vi "Monitoreo.vi"() -> ()   [LabVIEW 2020]
uses:
  <vilib>/Instr/_visa.llb/VISA Configure Serial Port (Instr).vi
panel:
  out "x+1":dbl
  out "concatenated string 2":string
  in  "string":string
  out "concatenated string":string
  in  "Boolean 2":bool
  in  "Boolean":bool
  in  "stop":bool
  in  "VISA resource name":refnum<visa-resource-name>
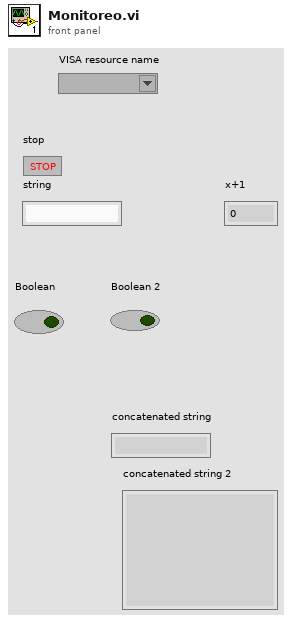
[diagram p1: front panel]
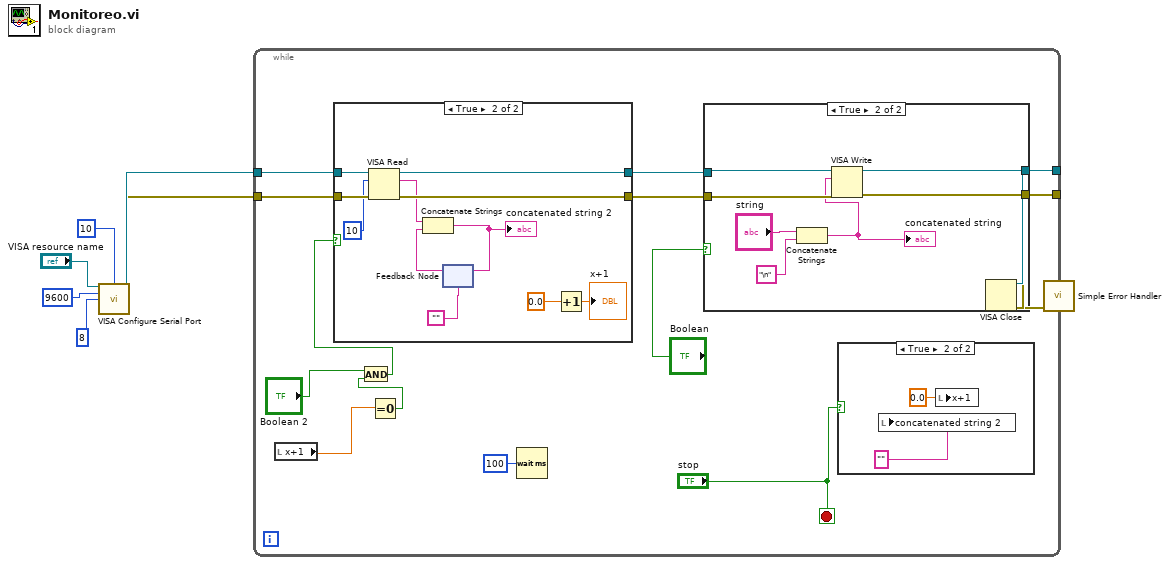
[diagram p0: block diagram]
diagram:
  n1 = call-poly "VISA Configure Serial Port"("VISA resource name"="VISA resource name", "termination char\n(0xA = '\\n' = LF)"=u8 10 ("termination char\n(0xA = '\\n' = LF)"), "baud rate (9600)"=u32 9600, "data bits (8)"=u16 8) -> ("VISA resource name out"=w7:refnum<visa-resource-name>, "error out"=w6:errorcluster)  [unwired: 10 in]
  n2 = while {
    tunnel: w7 -> [w22]
    tunnel: w6 -> [w17]
    tunnel: [w20] -> w5
    tunnel: [w18] -> w3
    stop <- "stop" stop-if-true
    n3 = local read "x+1"() -> (w13:dbl)
    n4 = Equal To 0?(x=w13) -> (x = 0?=w12:bool)
    n5 = And(x="Boolean 2", y=w12) -> (x .and. y?=w10:bool)
    n6 = case shown="True" w10 {
      tunnel: w22 -> [w35 w46]
      tunnel: [w35 w45] -> w21
      tunnel: [w34 w44] -> w19
      tunnel: w17 -> [w34 w40]
      frame False {
      }
      frame True {
        n7 = VISA Read(VISA resource name=w46, byte count=u32 10, error in (no error)=w40) -> (VISA resource name out=w45:refnum<visa-resource-name>, read buffer=w43:string, error out=w44:errorcluster)  [unwired: 1 out]
        n8 = feedback #1("") -> (w42:string)
        n9 = Concatenate Strings(w43, w42) -> (w38:string)
        "concatenated string 2" <- w38
        n10 = feedback-in #1(w38) -> ()
        n11 = Increment(x=0.0) -> (x+1=→"x+1":dbl)
      }
    }
    n12 = Wait (ms)(milliseconds to wait=u32 100) -> ()  [unwired: 1 out]
    n13 = case shown="True" "Boolean" {
      tunnel: w21 -> [w26 w33]
      tunnel: [w26 w32] -> w20
      tunnel: w19 -> [w25 w31]
      tunnel: [w25 w30] -> w18
      frame False {
      }
      frame True {
        n14 = Concatenate Strings("string", "\n" ("string")) -> (w27:string)
        "concatenated string" <- w27
        n15 = VISA Write(VISA resource name=w33, write buffer=w27, error in (no error)=w31) -> (VISA resource name out=w32:refnum<visa-resource-name>, error out=w30:errorcluster)  [unwired: 1 out]
      }
    }
    n16 = case shown="True" "stop" {
      frame False {
      }
      frame True {
        n17 = local write "concatenated string 2"("" ("concatenated string 2")) -> ()
        n18 = local write "x+1"(0.0 ("x+1")) -> ()
      }
    }
  }
  n19 = VISA Close(VISA resource name=w5, error in (no error)=w3) -> (error out=w1:errorcluster)
  n20 = call <vilib>:"Simple Error Handler.vi"("error in (no error)"=w1) -> ()  [unwired: 4 in, 5 out]
